vi "Add to Statistics.vi"(10 "Non Object":refnum<class "JSON Value.lvclass">, 11 "JSON Statistics in":refnum<class "JSON Statistics.lvclass">) -> (3 "JSON Statistics out":refnum<class "JSON Statistics.lvclass">)   [LabVIEW 2020, in "Library Commun.lvlib" / "JSON Statistics.lvclass"]
uses:
  JSON Statistics.lvclass
  JSON Value/JSON Value.lvclass
  JSON Statistics.lvclass/JSON Statistics.ctl
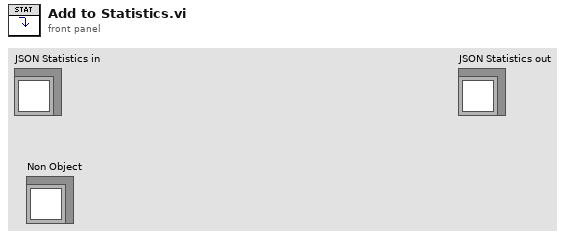
[diagram p1: front panel]
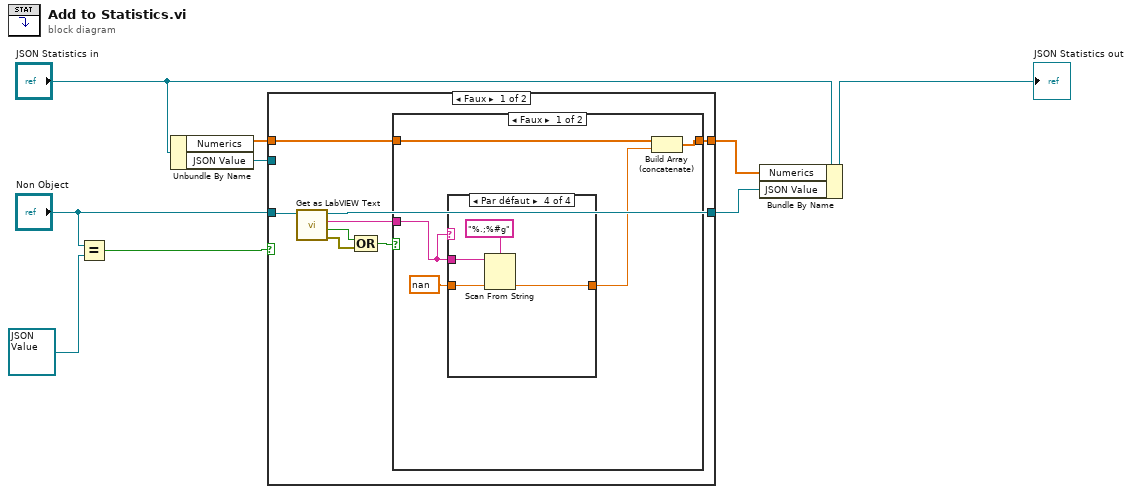
[diagram p0: block diagram]
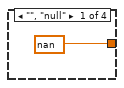
[diagram p2: hidden frame]
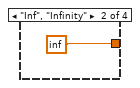
[diagram p3: hidden frame]
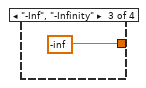
[diagram p4: hidden frame]
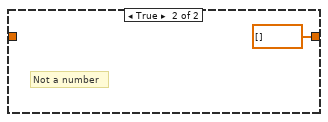
[diagram p5: hidden frame]
diagram:
  n1 = Equal?(x="Non Object", y=refnum<class "JSON Value.lvclass"> refnum) -> (x = y?=w4:bool)
  n2 = Unbundle By Name("JSON Statistics in") -> ("Numerics"=w7:sgl[], "JSON Value"=w1:refnum<class "JSON Value.lvclass">)
  n3 = case shown="Faux" w4 {
    tunnel: w7 -> [w17 w32]
    tunnel: [w16 w32] -> w6
    tunnel: "Non Object" -> [w15 _]
    tunnel: [w14 w31] -> w2
    tunnel: w1 -> [_ w31]
    frame False {
      n4 = call-dynamic "Get as LabVIEW Text.vi"("JSON Value In"=w15) -> ("error out"=w11:errorcluster, "Was in quotes"=w12:bool, "LabVIEW Text"=w13:string, "JSON Value Out"=w14:refnum<class "JSON Value.lvclass">)  [unwired: 7 in]
      n5 = Compound Arithmetic op=OR(w12, w11) -> (w10:bool)
      n6 = case shown="Faux" w10 {
        tunnel: w17 -> [w22 _]
        tunnel: [w21 sgl[] []] -> w16
        tunnel: w13 -> [w19 _]
        frame False {
          n7 = case shown="Par défaut" w19 {
            tunnel: [sgl nan ("default value 1") sgl inf ("default value 1") sgl -inf ("default value 1") w27] -> w18
            tunnel: sgl nan ("default value 1") -> [_ _ _ w29]
            tunnel: w19 -> [_ _ _ w28]
            frame "", "null" {
            }
            frame "Inf", "Infinity" {
            }
            frame "-Inf", "-Infinity" {
            }
            frame Default {
              n8 = Scan From String(format string="%.;%#g", input string=w28, default 1=w29) -> (output 1=w27:sgl)  [unwired: 2 in, 3 out]
            }
          }
          n9 = Build Array (concatenate)(w22, w18) -> (w21:sgl[])
        }
        frame True {
          # "Not a number"
        }
      }
    }
    frame True {
    }
  }
  n10 = Bundle By Name(cluster="JSON Statistics in", "Numerics"=w6, "JSON Value"=w2) -> (→"JSON Statistics out":refnum<class "JSON Statistics.lvclass">)
